vi "dll.midi_send_message.vi"(8 "error in (no error)":errorcluster, 10 "message array (U8)":u8[](array[numeric]), 11 "midi out in":refnum<class "midi out.lvclass">) -> (0 "error out":errorcluster, 3 "midi out":refnum<class "midi out.lvclass">)   [LabVIEW 2020, in "midi out.lvclass"]
uses:
  midi out.lvclass
  midi out.lvclass/midi out.ctl
  shared/midi shared.lvlib
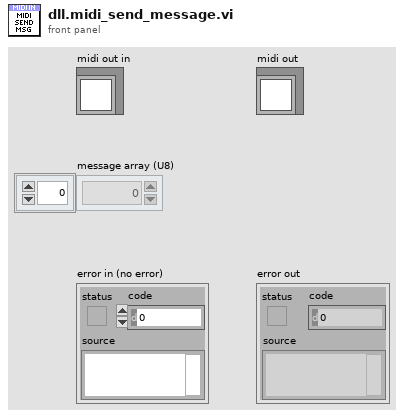
[diagram p1: front panel]
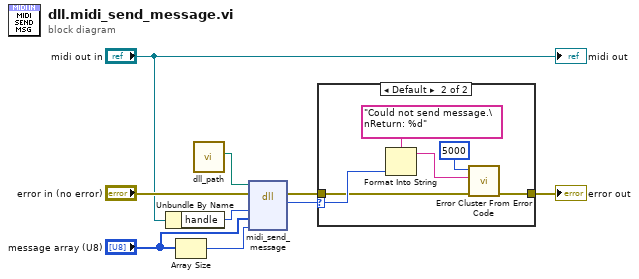
[diagram p0: block diagram]
diagram:
  n1 = Unbundle By Name("midi out in") -> ("handle"=w6:i32)
  n2 = Array Size(array="message array (U8)") -> (size(s)=w4:i32)
  n3 = call "dll_path.vi"() -> ("dll"=w8:path)  [unwired: 11 in]
  n4 = dll-call lib="C:/code/LabVIEW-MIDI-XPLAT/dist/TomMIDIllan_*.*" fn="midi_send_message"(path in=w8, error in="error in (no error)", "manager_handle"=w6, "message_array"="message array (U8)", "message_length"=w4) -> (error out=w2:errorcluster, "return type"=w3:i32)  [unwired: 4 in, 1 out]
  n5 = case shown="Default" w3 {
    selector: w3 -> [_ w13]
    tunnel: w2 -> [w10 w12]
    tunnel: [w10 w11] -> w1
    frame 0.. {
    }
    frame Default {
      n6 = Format Into String(format string="Could not send message.\nReturn: %d", w13) -> (resulting string=w14:string)  [unwired: 2 in, 1 out]
      n7 = call <vilib>:"Error Cluster From Error Code.vi"("error in (no error)"=w12, "error message (\"\")"=w14, "error code (0)"=5000) -> ("error out"=w11:errorcluster)  [unwired: 6 in]
    }
  }
  "error out" <- w1
  "midi out" <- "midi out in"
